vi "rs3_close all.vi"(6 "rscontext":u64, 7 "queue in":u64, 8 "error in (no error)":errorcluster, 9 "device_list":u64, 10 "Dev in":u64, 11 "Sensor in":u64) -> (0 "error out (no error)":errorcluster, 3 "Close Error":string)   [LabVIEW 2017, in "libRealSense3.lvlib"]
doc: "It is important to close everything properly at the end. Use this VI to clean up and close the RealSense device, queue, sensor, and device list."
uses:
  <vilib>/addons/RealSense/libRealSense3.lvlib
panel:
  # "RS3 Close All"
  # "(C) Intel Corp. 2017,  AGJ"
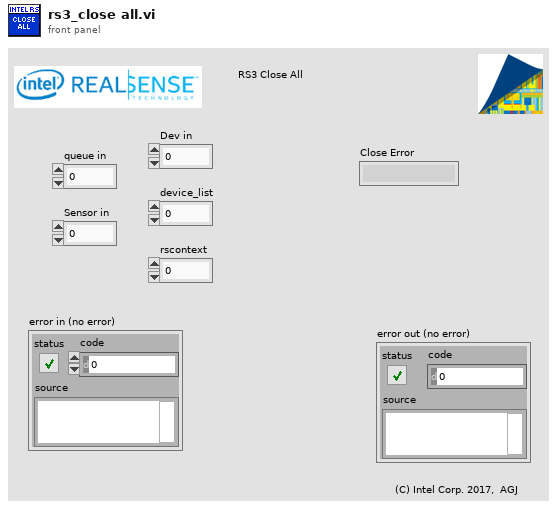
[diagram p1: front panel]
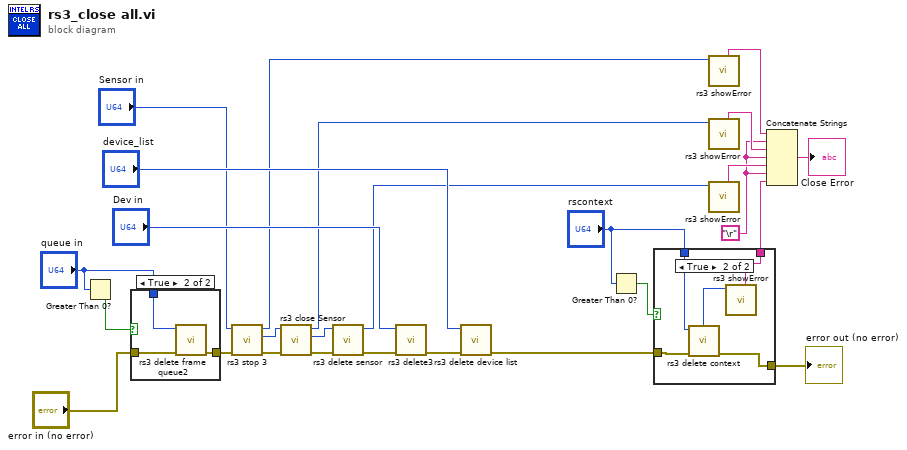
[diagram p0: block diagram]
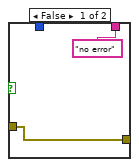
[diagram p3: hidden frame]
diagram:
  w7 = "\r"
  n1 = Greater Than 0?(x="queue in") -> (x > 0?=w3:bool)
  n2 = case shown="True" w3 {
    tunnel: "error in (no error)" -> [w27 w30]
    tunnel: "queue in" -> [_ w29]
    tunnel: [w27 w28] -> w11
    frame False {
    }
    frame True {
      n3 = call <vilib>:"rs3 delete frame queue2.vi"("error in (no error)"=w30, "queue"=w29) -> ("error out"=w28:errorcluster)  [unwired: 9 in]
    }
  }
  n4 = call <vilib>:"rs3 stop 3.vi"("error in (no error)"=w11, "sensor"="Sensor in") -> ("error out"=w10:errorcluster, "sensor out"=w8:u64, "error"=w5:u64)  [unwired: 7 in]
  n5 = call <vilib>:"rs3 close Sensor.vi"("error in (no error)"=w10, "sensor"=w8) -> ("error out"=w24:errorcluster, "device out"=w23:u64, "error"=w14:u64)  [unwired: 7 in]
  n6 = call <vilib>:"rs3 delete sensor.vi"("error in (no error)"=w24, "sensor"=w23) -> ("error out"=w25:errorcluster, "error"=w13:u64)  [unwired: 8 in]
  n7 = call <vilib>:"rs3 delete3.vi"("error in (no error)"=w25, "device"="Dev in") -> ("error out"=w20:errorcluster)  [unwired: 9 in]
  n8 = call <vilib>:"rs3 delete device list.vi"("error in (no error)"=w20, "device list"="device_list") -> ("error out"=w22:errorcluster)  [unwired: 9 in]
  n9 = Greater Than 0?(x="rscontext") -> (x > 0?=w1:bool)
  n10 = case shown="True" w1 {
    tunnel: w22 -> [w31 w37]
    tunnel: [w31 w36] -> w18
    tunnel: ["no error" ("Error summary") w34] -> w12
    tunnel: "rscontext" -> [_ w33]
    frame False {
    }
    frame True {
      n11 = call <vilib>:"rs3 delete context.vi"("error in (no error)"=w37, "context"=w33) -> ("error out"=w36:errorcluster, "error"=w35:u64)  [unwired: 8 in]
      n12 = call <vilib>:"rs3 showError.vi"("error"=w35) -> ("Error summary"=w34:string)  [unwired: 6 in, 4 out]
    }
  }
  "error out (no error)" <- w18
  n13 = call <vilib>:"rs3 showError.vi"("error"=w5) -> ("Error summary"=w6:string)  [unwired: 6 in, 4 out]
  n14 = call <vilib>:"rs3 showError.vi"("error"=w14) -> ("Error summary"=w17:string)  [unwired: 6 in, 4 out]
  n15 = call <vilib>:"rs3 showError.vi"("error"=w13) -> ("Error summary"=w16:string)  [unwired: 6 in, 4 out]
  n16 = Concatenate Strings(w6, w7, w17, w7, w16, w7, w12) -> (→"Close Error":string)
